vi "Hall.vi"() -> ()   [LabVIEW 2018]
panel:
  in  "Flatness":dbl=0.05
  out "R Hall mean":dbl
  out "XY Graph 2":cluster{"Field":dbl[], dbl[]}[](graph)
  in  "Bin size":dbl=0.1
  out "XY Graph":cluster{dbl[], dbl[]}[](graph)
  in  "Signal channel":string="LakeShore 370 (20) R"
  in  "Field channel":string="IPS120 (25) Field"
  in  "Group":string="p"
  in  "File Path Control":path
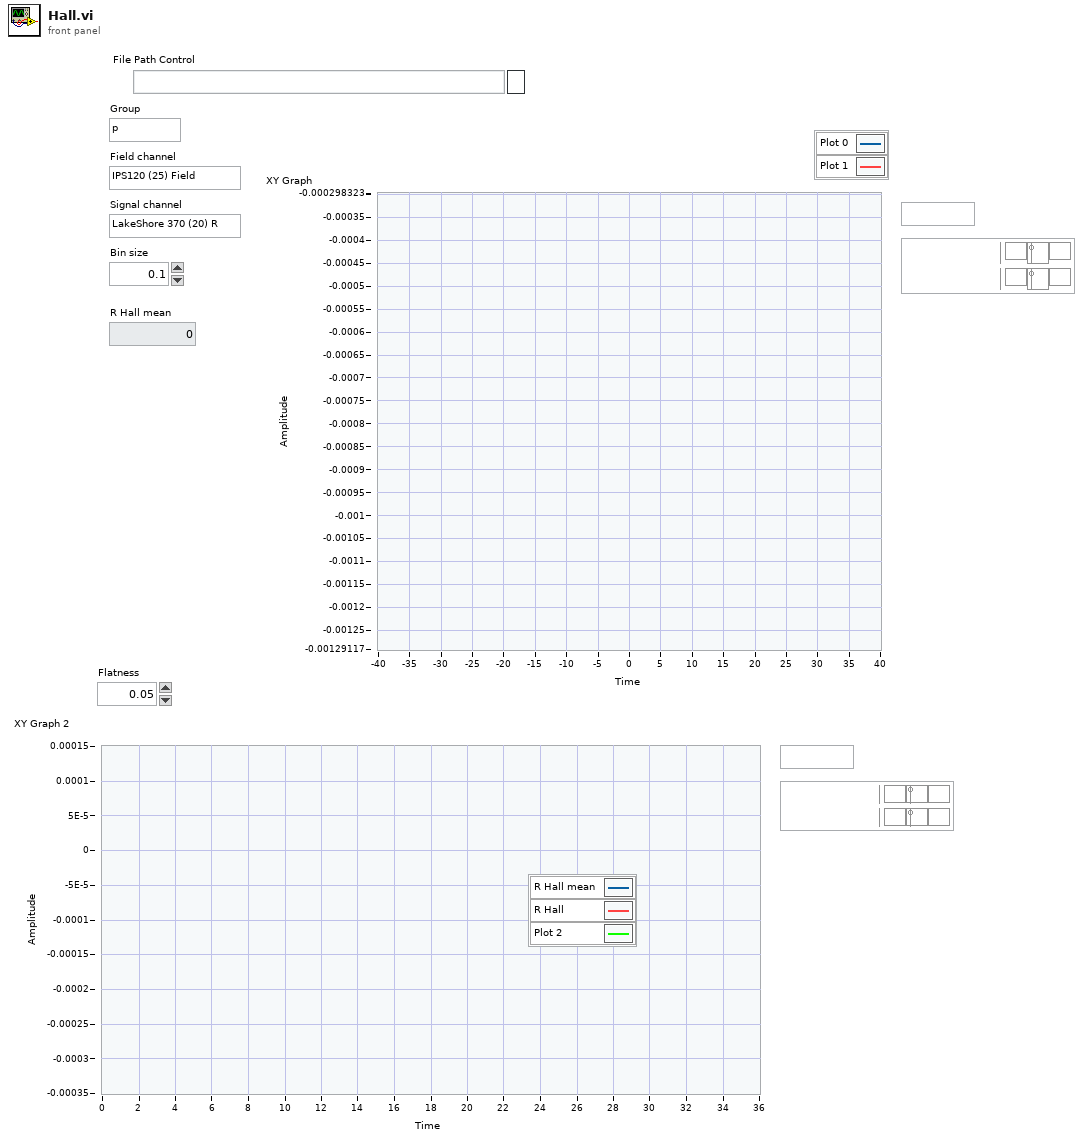
[diagram p1: front panel]
types:
  T1 = enum16{"open", "open or create", "create or replace", "create", "open (read-only)"}
  T2 = cluster{"Binned data":dbl[], "Binned data":dbl[]}
  T3 = cluster{"Binned data":dbl[], "Binned data":dbl[]}[]
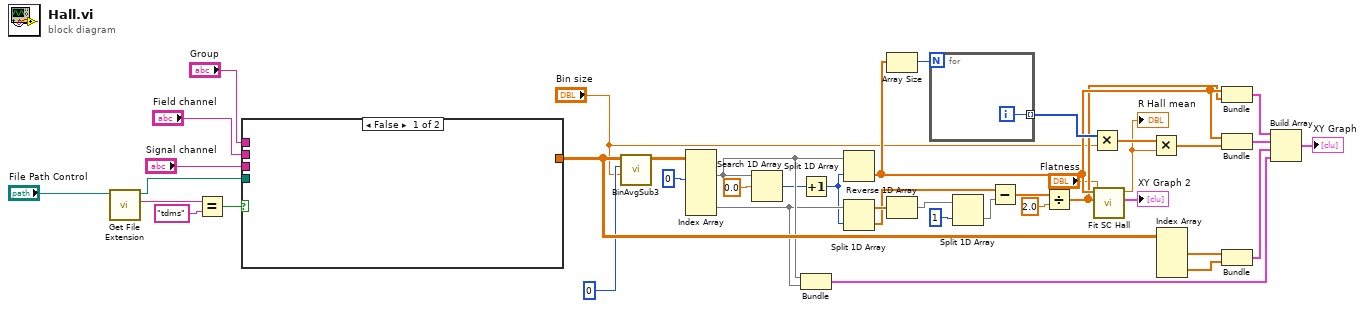
[diagram p0: block diagram]
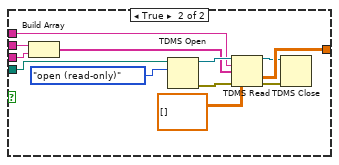
[diagram p2: hidden frame]
diagram:
  n1 = call <vilib>:"Get File Extension.vi"("file"="File Path Control") -> ("lowercase file extension"=w4:string, "dup file"=w5:path)  [unwired: 6 in, 3 out]
  n2 = Equal?(x=w4, y="tdms") -> (x = y?=w2:bool)
  n3 = case shown="False" w2 {
    tunnel: w5 -> [_ w53]
    tunnel: "Group" -> [_ w49]
    tunnel: "Field channel" -> [_ w48]
    tunnel: "Signal channel" -> [_ w46]
    tunnel: [_ w44] -> w35
    frame False {
    }
    frame True {
      n4 = Build Array(w48, w46) -> (w47:string[])
      n5 = TDMS Open(10:T1."open (read-only)" ("operation (0:open)"), 11:w53) -> (0:w50:errorcluster, 3:w51:refnum<k34>)  [unwired: 5 in]
      n6 = TDMS Read(0:w51, 5:w49, 7:w47, 11:w50, 12:dbl[][] []) -> (4:w42:refnum<k34>, 10:w44:dbl[][], 15:w43:errorcluster)  [unwired: 3 in, 3 out]
      n7 = TDMS Close(8:w43, 11:w42) -> ()  [unwired: 2 out]
    }
  }
  n8 = call "BinAvgSub3.vi"("Bin size"="Bin size", "X coumn index"=0, "Data in"=w35) -> ("Binned data"=w32:dbl[][])  [unwired: 2 in, 6 out]
  n9 = Index Array(array=w32, index (col) #1=0 ("disabled index (col)")) -> (element #1=w28:dbl[], element #3=w26:dbl[])  [unwired: 5 in, 1 out]
  n10 = Search 1D Array(1D array=w28, element=0.0) -> (index of element=w27:i32)  [unwired: 1 in]
  n11 = Increment(x=w27) -> (x+1=w25:i32)
  n12 = Bundle("Binned data"=w28, "Binned data"=w26) -> (w31:T2)  [unwired: 1 in]
  n13 = Split 1D Array(array=w28, index=w25) -> (second subarray=w14:dbl[])  [unwired: 1 out]
  n14 = Split 1D Array(array=w26, index=w25) -> (first subarray=w24:dbl[], second subarray=w21:dbl[])
  n15 = Array Size(array=w14) -> (size(s)=w19:i32)
  n16 = Reverse 1D Array(array=w24) -> (reversed array=w23:dbl[])
  n17 = for {
    N: w19 -> [_]
    tunnel: [w54] -> w18 mode=indexing
    i -> [w54]
  }
  n18 = Split 1D Array(array=w23, index=1) -> (second subarray=w20:dbl[])  [unwired: 1 out]
  n19 = Subtract(x=w21, y=w20) -> (x-y=w12:dbl[])
  n20 = Divide(x=w12, y=2.0) -> (x/y=w13:dbl[])
  n21 = Multiply(x=w18, y="Bin size") -> (x*y=w9:dbl[])
  n22 = call "Fit SC Hall.vi"("Flatness"="Flatness", "Hall signal"=w13, "Field"=w14) -> ("XY Graph"=→"XY Graph 2":cluster{"Field":dbl[], dbl[]}[], "Mean"=w7:dbl)  [unwired: 7 in]
  "R Hall mean" <- w7
  n23 = Multiply(x=w9, y=w7) -> (x*y=w15:dbl[])
  n24 = Index Array(array=w35) -> (element #1=w37:dbl[], element #2=w36:dbl[])  [unwired: 4 in]
  n25 = Bundle(w14, w13) -> (w17:cluster{dbl[], dbl[]})  [unwired: 1 in]
  n26 = Bundle(w14, w15) -> (w16:cluster{dbl[], dbl[]})  [unwired: 1 in]
  n27 = Bundle(w37, w36) -> (w39:cluster{dbl[], dbl[]})  [unwired: 1 in]
  n28 = Build Array(w17, w16, w39, w31) -> (→"XY Graph":T3)
